vi "quack.vi"(8 "error in (no error)":errorcluster, 11 "MuteQuack in":refnum<class "MuteQuack.lvclass">) -> (0 "error out":errorcluster, 2 "String":string, 3 "MuteQuack out":refnum<class "MuteQuack.lvclass">)   [LabVIEW 2013, in "MuteQuack.lvclass"]
uses:
  MuteQuack.lvclass
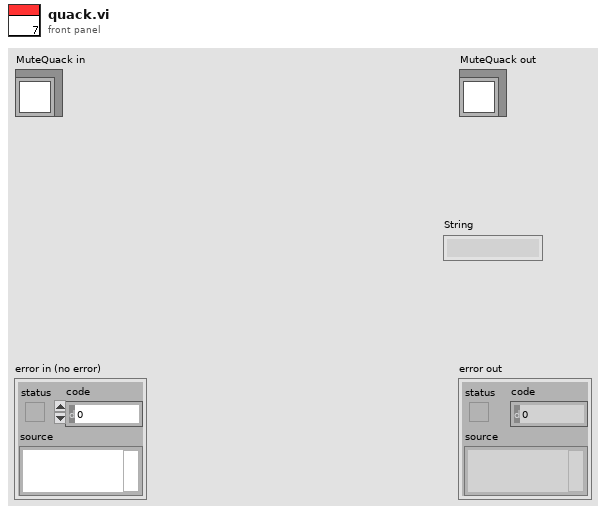
[diagram p1: front panel]
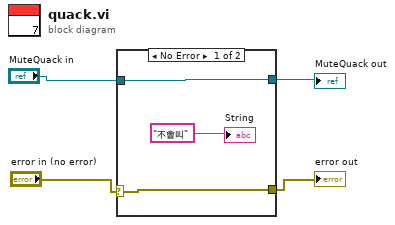
[diagram p0: block diagram]
diagram:
  n1 = case shown="No Error" "error in (no error)" {
    selector: "error in (no error)" -> [w7 w9]
    tunnel: [w7 w9] -> w2
    tunnel: [w6 w8] -> w1
    tunnel: "MuteQuack in" -> [w6 w8]
    frame No Error {
      "String" <- "不會叫" ("String")
    }
    frame Error {
    }
  }
  "error out" <- w2
  "MuteQuack out" <- w1
